vi "publishJobUpdate.vi"(8 "error in (no error)":errorcluster, 9 "% Complete (NaN if unknown)":dbl=nan, 10 "Status Message":string, 11 "Job in":refnum<class "Job.lvclass">) -> (0 "error out":errorcluster, 3 "Job out":refnum<class "Job.lvclass">)   [LabVIEW 2013, in "openCronJob.lvlib" / "Job.lvclass"]
uses:
  Job.lvclass
  Job Update -- cluster.ctl
  Job.lvclass/Job.ctl
  JobReport/JobReport.lvclass
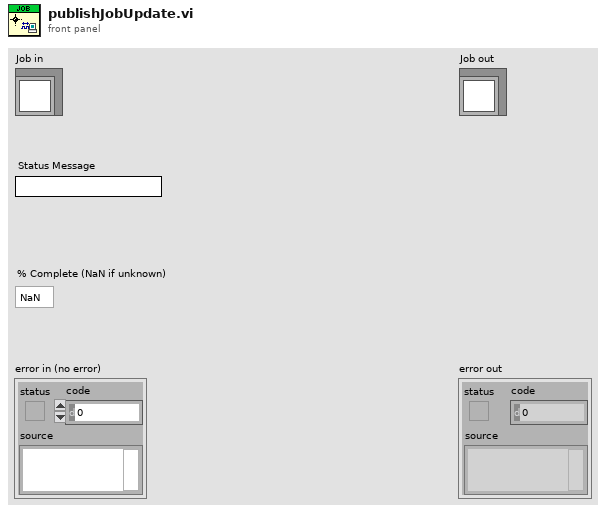
[diagram p1: front panel]
types:
  T1 = typedef "openCronJob.lvlib/Job.lvclass/Job Update -- cluster.ctl" = cluster{"Name":string, "GUID":string, "Time Stamp":timestamp, "Status Message":string, "% Complete":dbl}
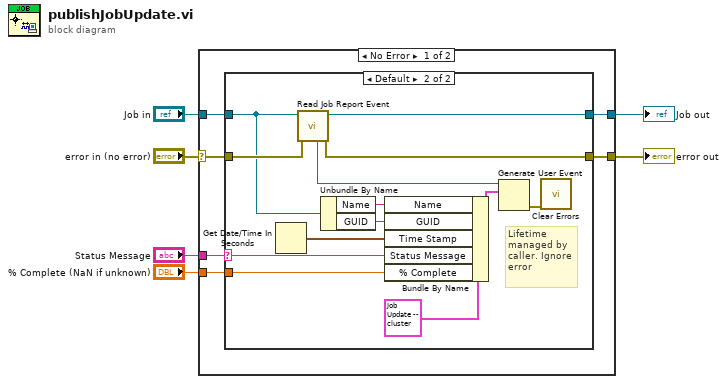
[diagram p0: block diagram]
diagram:
  n1 = case shown="No Error" "error in (no error)" {
    selector: "error in (no error)" -> [w11 w29]
    tunnel: [w10 w29] -> w5
    tunnel: [w9 w28] -> w3
    tunnel: "Job in" -> [w8 w28]
    tunnel: "Status Message" -> [w7 _]
    tunnel: "% Complete (NaN if unknown)" -> [w12 _]
    frame No Error {
      n2 = case shown="Default" w7 {
        selector: w7 -> [_ w18]
        tunnel: w12 -> [_ w19]
        tunnel: w11 -> [w13 w26]
        tunnel: [w13 w24] -> w10
        tunnel: [w14 w27] -> w9
        tunnel: w8 -> [w14 w22]
        frame "" {
        }
        frame Default {
          # "Lifetime\nmanaged by\ncaller. Ignore\nerror"
          n3 = Get Date/Time In Seconds() -> (seconds since 1Jan1904=w15:timestamp)
          n4 = call "Read Job Report Event.vi"("error in (no error)"=w26, "Job in"=w22) -> ("error out"=w24:errorcluster, "Job out"=w27:refnum<class "Job.lvclass">, "Job Update Event"=w25:refnum<user-event>)  [unwired: 5 in, 2 out]
          n5 = Unbundle By Name(w22) -> ("Name"=w20:string, "GUID"=w17:string)
          n6 = Bundle By Name(cluster=T1 {"Name"="", "GUID"="", "Time Stamp"=timestamp(0 s since 1904-01-01), "Status Message"="", "% Complete"=nan} ("Job Update"), "Name"=w20, "GUID"=w17, "Time Stamp"=w15, "Status Message"=w18, "% Complete"=w19) -> (w16:T1)
          n7 = Generate User Event(user event=w25, event data cluster=w16) -> (error out=w23:errorcluster)  [unwired: 2 in, 1 out]
          n8 = call <vilib>:"Clear Errors.vi"("error in (no error)"=w23) -> ()  [unwired: 6 in, 1 out]
        }
      }
    }
    frame Error {
    }
  }
  "error out" <- w5
  "Job out" <- w3
